vi "status.vi"(3 "error in (no error)":errorcluster, 5 "HGF_Monitor in":refnum<class "HGF_Monitor.lvclass">) -> (0 "error out":errorcluster, 1 "Array":T1(array[cluster]), 2 "HGF_Monitor out":refnum<class "HGF_Monitor.lvclass">)   [LabVIEW 2012, in "HGF_SV.lvlib" / "HGF_Monitor.lvclass"]
uses:
  HGF_Monitor.lvclass
  HGF_BaseClasses/HGF_NetworkVisitor/HGF_NetworkVisitor.lvclass
  HGF_BaseClasses/HGF_TriggeredEvent/HGF_TriggeredEvent.lvclass
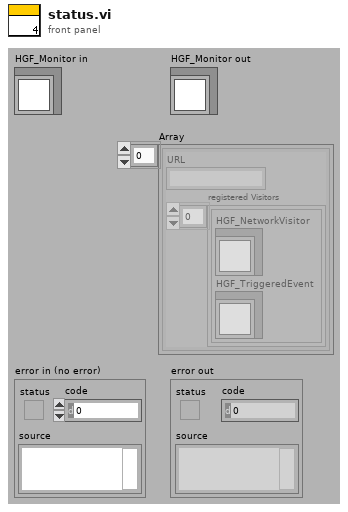
[diagram p1: front panel]
types:
  T1 = cluster{"URL":string, "registered Visitors":cluster{"HGF_NetworkVisitor":refnum<class "HGF_NetworkVisitor.lvclass">, "HGF_TriggeredEvent":refnum<class "HGF_TriggeredEvent.lvclass">}[]}[]
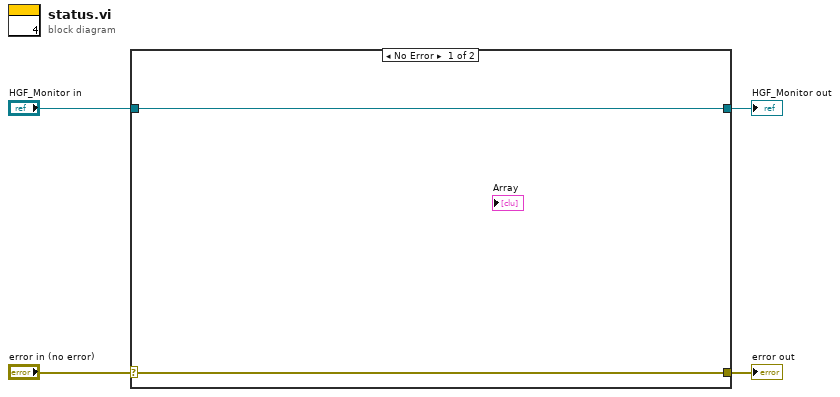
[diagram p0: block diagram]
diagram:
  n1 = case shown="No Error" "error in (no error)" {
    selector: "error in (no error)" -> [w5 w8]
    tunnel: [w5 w8] -> w3
    tunnel: [w6 w7] -> w1
    tunnel: "HGF_Monitor in" -> [w6 w7]
    frame No Error {
    }
    frame Error {
    }
  }
  "error out" <- w3
  "HGF_Monitor out" <- w1
